vi "4psk.vi"() -> ()   [LabVIEW 2014]
uses:
  <vilib>/Analysis/NI_AALPro.lvlib
panel:
  out "Demodulated":dynamicdata(graph)
  out "modulated":dynamicdata(graph)
  out "dig.data":dbl[](graph)
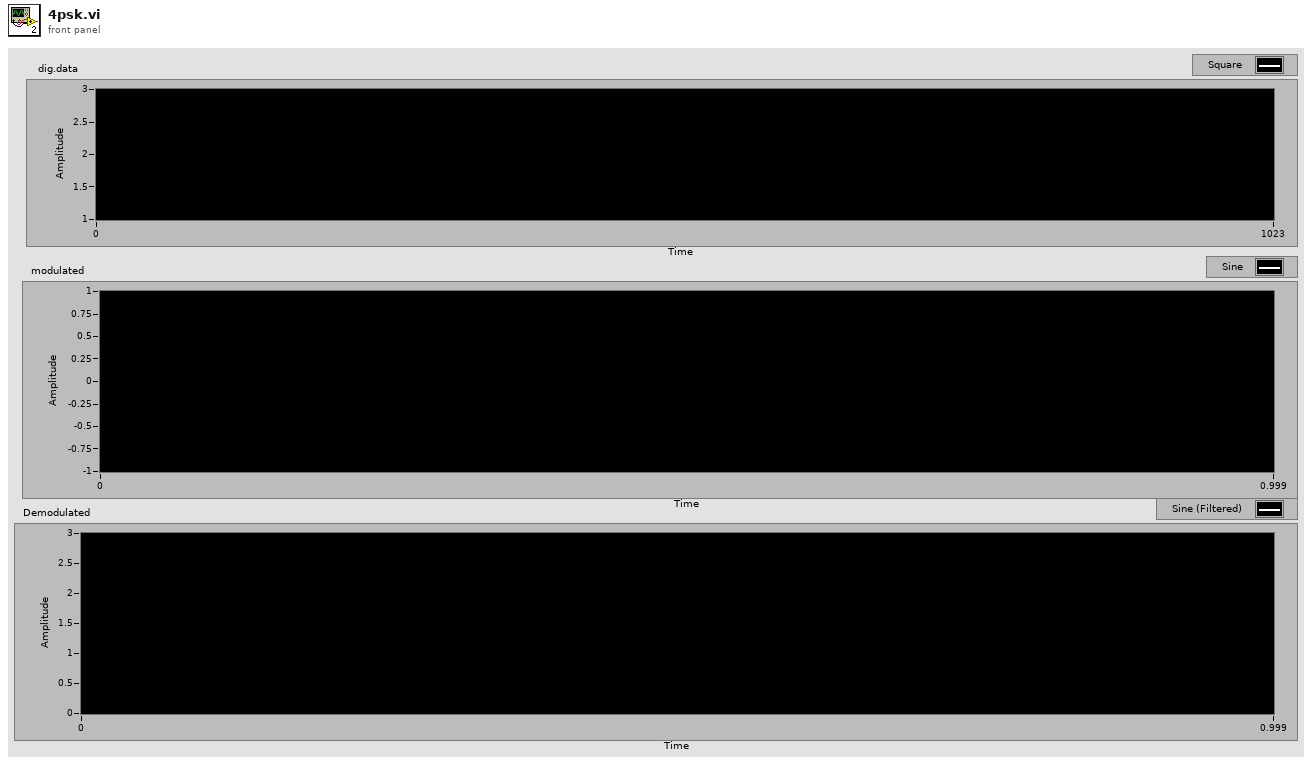
[diagram p1: front panel]
types:
  T1 = enum16{"sine", "cosine", "triangle", "square", "sawtooth", "increasing ramp", "decreasing ramp"}
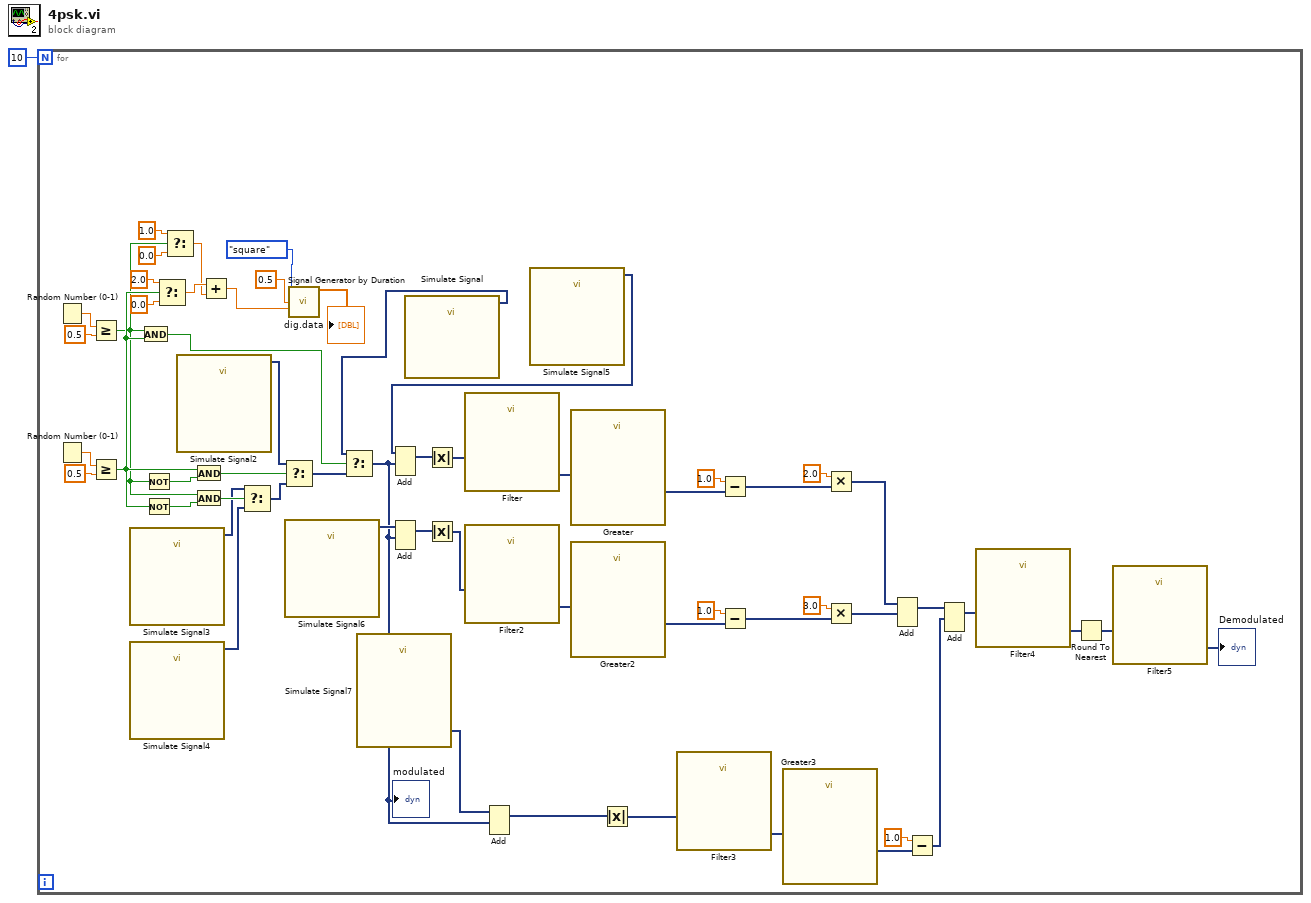
[diagram p0: block diagram]
diagram:
  n1 = for {
    N: 10 -> [_]
    n2 = Random Number (0-1)() -> (number: 0 to 1=w57:dbl)
    n3 = Random Number (0-1)() -> (number: 0 to 1=w59:dbl)
    n4 = Greater Or Equal?(x=w57, y=0.5) -> (x >= y?=w37:bool)
    n5 = Greater Or Equal?(x=w59, y=0.5) -> (x >= y?=w38:bool)
    n6 = call "Simulate Signal3"() -> ("Sine"=w35:dynamicdata)  [unwired: 14 in, 1 out]
    n7 = call "Simulate Signal4"() -> ("Sine"=w34:dynamicdata)  [unwired: 14 in, 1 out]
    n8 = And(x=w37, y=w38) -> (x .and. y?=w44:bool)
    n9 = Not(x=w37) -> (.not. x?=w42:bool)
    n10 = Not(x=w38) -> (.not. x?=w39:bool)
    n11 = Select(t=2.0, s=w38, f=0.0) -> (s? t:f=w51:dbl)
    n12 = Select(t=1.0, s=w37, f=0.0) -> (s? t:f=w50:dbl)
    n13 = call "Simulate Signal2"() -> ("Sine"=w40:dynamicdata)  [unwired: 14 in, 1 out]
    n14 = And(x=w38, y=w42) -> (x .and. y?=w41:bool)
    n15 = And(x=w37, y=w39) -> (x .and. y?=w36:bool)
    n16 = Add(x=w51, y=w50) -> (x+y=w46:dbl)
    n17 = Select(t=w35, s=w36, f=w34) -> (s? t:f=w33:dynamicdata)
    n18 = Select(t=w40, s=w41, f=w33) -> (s? t:f=w43:dynamicdata)
    n19 = call "Simulate Signal6"() -> ("Sine"=w28:dynamicdata)  [unwired: 14 in, 1 out]
    n20 = call <vilib>:"Signal Generator by Duration.vi"("signal type"=T1."square", "frequency"=0.5, "amplitude"=w46) -> ("signal"=→"dig.data":dbl[])  [unwired: 9 in, 3 out]
    n21 = call "Simulate Signal7"() -> ("Sine"=w15:dynamicdata)  [unwired: 14 in, 1 out]
    n22 = call "Simulate Signal"() -> ("Sine"=w45:dynamicdata)  [unwired: 14 in, 1 out]
    n23 = Select(t=w45, s=w44, f=w43) -> (s? t:f=w16:dynamicdata)
    "modulated" <- w16
    n24 = Add(1:w16, 2:w28) -> (0:w27:dynamicdata)  [unwired: 1 in, 1 out]
    n25 = Absolute Value(x=w27) -> (abs(x)=w29:dynamicdata)
    n26 = call "Filter2"("Signal"=w29) -> ("Filtered Signal"=w30:dynamicdata)  [unwired: 9 in, 1 out]
    n27 = Add(1:w16, 2:w15) -> (0:w19:dynamicdata)  [unwired: 1 in, 1 out]
    n28 = call "Simulate Signal5"() -> ("Sine"=w24:dynamicdata)  [unwired: 14 in, 1 out]
    n29 = Add(1:w16, 2:w24) -> (0:w10:dynamicdata)  [unwired: 1 in, 1 out]
    n30 = Absolute Value(x=w10) -> (abs(x)=w31:dynamicdata)
    n31 = call "Filter"("Signal"=w31) -> ("Filtered Signal"=w32:dynamicdata)  [unwired: 9 in, 1 out]
    n32 = call "Greater"("Operand 1"=w32) -> ("Result"=w22:dynamicdata)  [unwired: 9 in, 1 out]
    n33 = call "Greater2"("Operand 1"=w30) -> ("Result"=w25:dynamicdata)  [unwired: 9 in, 1 out]
    n34 = Absolute Value(x=w19) -> (abs(x)=w20:dynamicdata)
    n35 = call "Filter3"("Signal"=w20) -> ("Filtered Signal"=w21:dynamicdata)  [unwired: 9 in, 1 out]
    n36 = Subtract(x=1.0, y=w22) -> (x-y=w14:dynamicdata)
    n37 = Subtract(x=1.0, y=w25) -> (x-y=w12:dynamicdata)
    n38 = call "Greater3"("Operand 1"=w21) -> ("Result"=w17:dynamicdata)  [unwired: 9 in, 1 out]
    n39 = Multiply(x=2.0, y=w14) -> (x*y=w9:dynamicdata)
    n40 = Multiply(x=3.0, y=w12) -> (x*y=w8:dynamicdata)
    n41 = Add(1:w8, 2:w9) -> (0:w7:dynamicdata)  [unwired: 1 in, 1 out]
    n42 = Subtract(x=1.0, y=w17) -> (x-y=w6:dynamicdata)
    n43 = Add(1:w6, 2:w7) -> (0:w5:dynamicdata)  [unwired: 1 in, 1 out]
    n44 = call "Filter4"("Signal"=w5) -> ("Filtered Signal"=w4:dynamicdata)  [unwired: 9 in, 1 out]
    n45 = Round To Nearest(number=w4) -> (nearest integer value=w3:dynamicdata)
    n46 = call "Filter5"("Signal"=w3) -> ("Filtered Signal"=→"Demodulated":dynamicdata)  [unwired: 9 in, 1 out]
  }
